vi "全局 环境参数.vi"() -> ()   [LabVIEW 2016]
panel:
  in  "湿度":string[][](array[string])
  in  "室温":string[][](array[string])
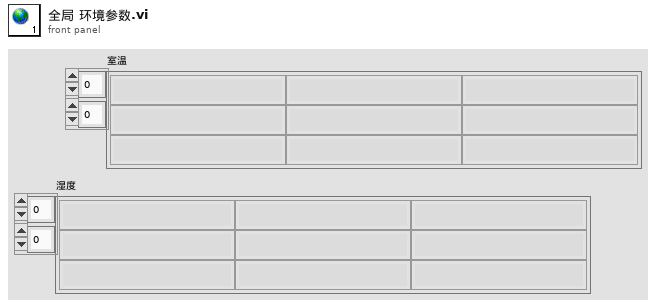
[diagram p1: front panel]
diagram:
